vi "serial_clear_reset_wait.vi"(2 "error in (no error)":errorcluster, 3 "VISA Refnum in":refnum<visa-resource-name>) -> (0 "error out":errorcluster, 1 "VISA Refnum out":refnum<visa-resource-name>)   [LabVIEW 2018]
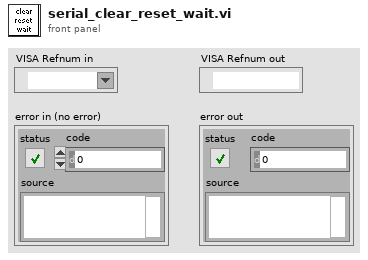
[diagram p1: front panel]
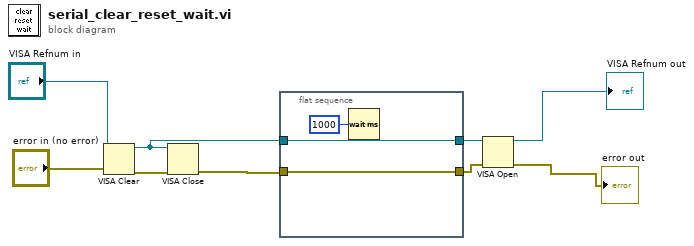
[diagram p0: block diagram]
diagram:
  n1 = VISA Clear(VISA resource name="VISA Refnum in", error in (no error)="error in (no error)") -> (VISA resource name out=w2:refnum<visa-resource-name>, error out=w7:errorcluster)
  n2 = VISA Close(VISA resource name=w2, error in (no error)=w7) -> (error out=w6:errorcluster)
  n3 = flat-sequence {
    tunnel: w6 -> [w11]
    tunnel: [w11] -> w5
    tunnel: [w10] -> w3
    tunnel: w2 -> [w10]
    frame #0 {
      n4 = Wait (ms)(milliseconds to wait=u32 1000) -> ()  [unwired: 1 out]
    }
  }
  n5 = VISA Open(error in (no error)=w5, VISA resource name=w3) -> (VISA resource name=→"VISA Refnum out":refnum<visa-resource-name>, error out=→"error out":errorcluster)  [unwired: 3 in]
